vi "op_num_v4.vi"() -> ()   [LabVIEW 2009]
panel:
  out "Waveform Chart":dbl(graph)
  out "N: numar aleator":dbl format="%.3f"
  out "Afisor numeric":i32
  # "- se genereaza un numar aleator N (valoarea lui N este cuprinsa intre 0-1)\n- se calculeaza produsul  N*1000 \n- se face o intarziere de 500 ms\n- se afiseaza rezultatul atat intr-un indicator numeric \n- se reprezinta grafic valorile calculate folosind un indicator de tip \"Waveform Chart\""
  # "Produsul N*1000 este:"
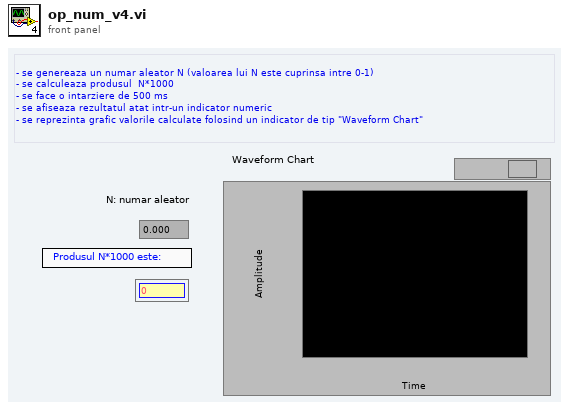
[diagram p1: front panel]
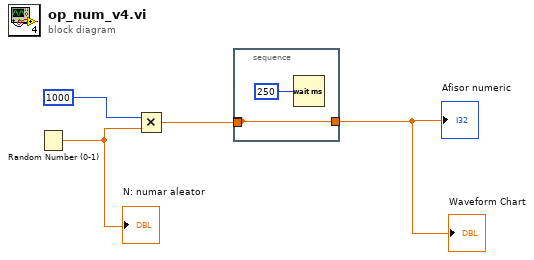
[diagram p0: block diagram]
diagram:
  n1 = Random Number (0-1)() -> (number: 0 to 1=w3:dbl)
  "N: numar aleator" <- w3
  n2 = Multiply(x=1000, y=w3) -> (x*y=w2:dbl)
  n3 = stacked-sequence {
    tunnel: [w5] -> _
    tunnel: w2 -> [w5]
    tunnel: [w5] -> w1
    frame #0 {
      n4 = Wait (ms)(milliseconds to wait=250) -> ()  [unwired: 1 out]
    }
  }
  "Afisor numeric" <- w1
  "Waveform Chart" <- w1
